vi "keyboardInput.vi"() -> ()   [LabVIEW 2023]
uses:
  <vilib>/regexp/Match Regular Expression.xnode
panel:
  out "Waveform Chart":dbl(graph)
  in  "MAIN STOP":bool
  out "data out 2":string
  out "code 2":i32
  in  "stop 4":bool
  out "Ostatnia 2":string
  out "PID":string
  in  "stop":bool
  in  "stop 3":bool
  out "code":i32
  out "Ostatnia":string
  out "data out":string
  in  "stop 2":bool
  out "ASCII Char 2":i16
  out "Character 2":string
  out "standard output 2":string
  out "standard output":string
  out "Character":string
  out "ASCII Char":i16
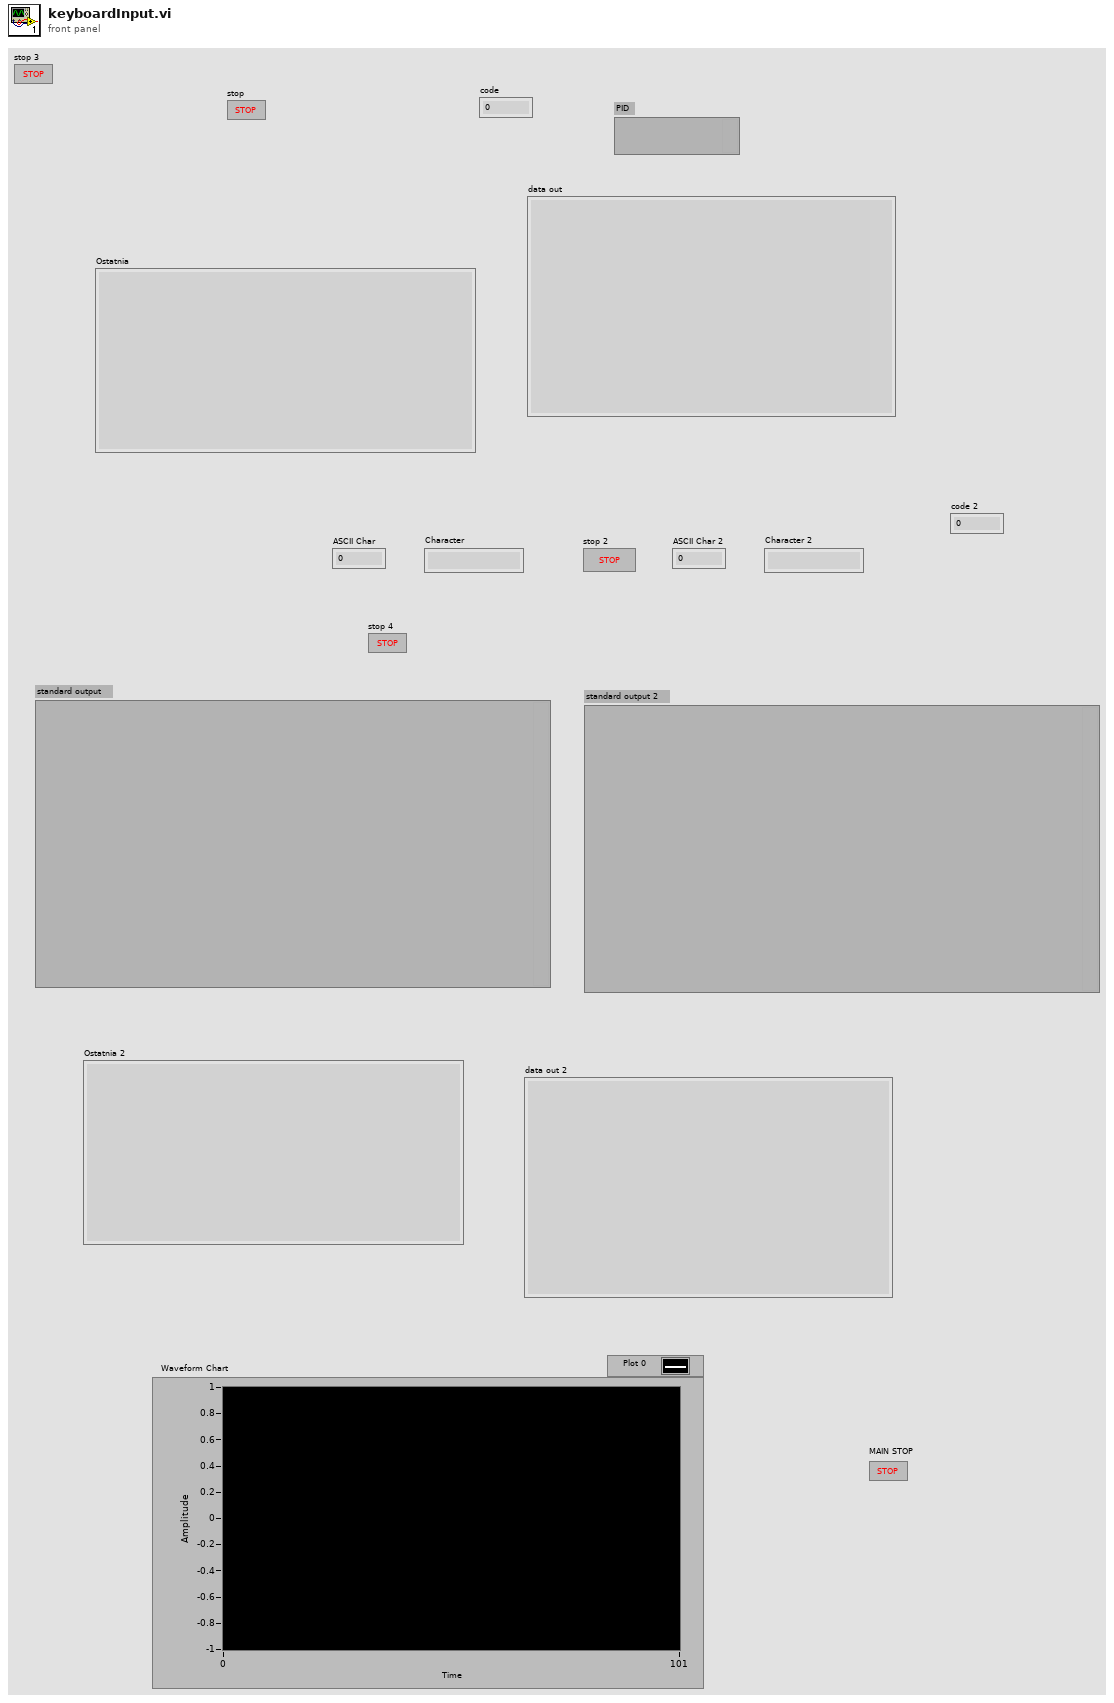
[diagram p1: front panel]
types:
  T1 = enum16{"Standard", "Buffered", "CRLF", "Immediate"}
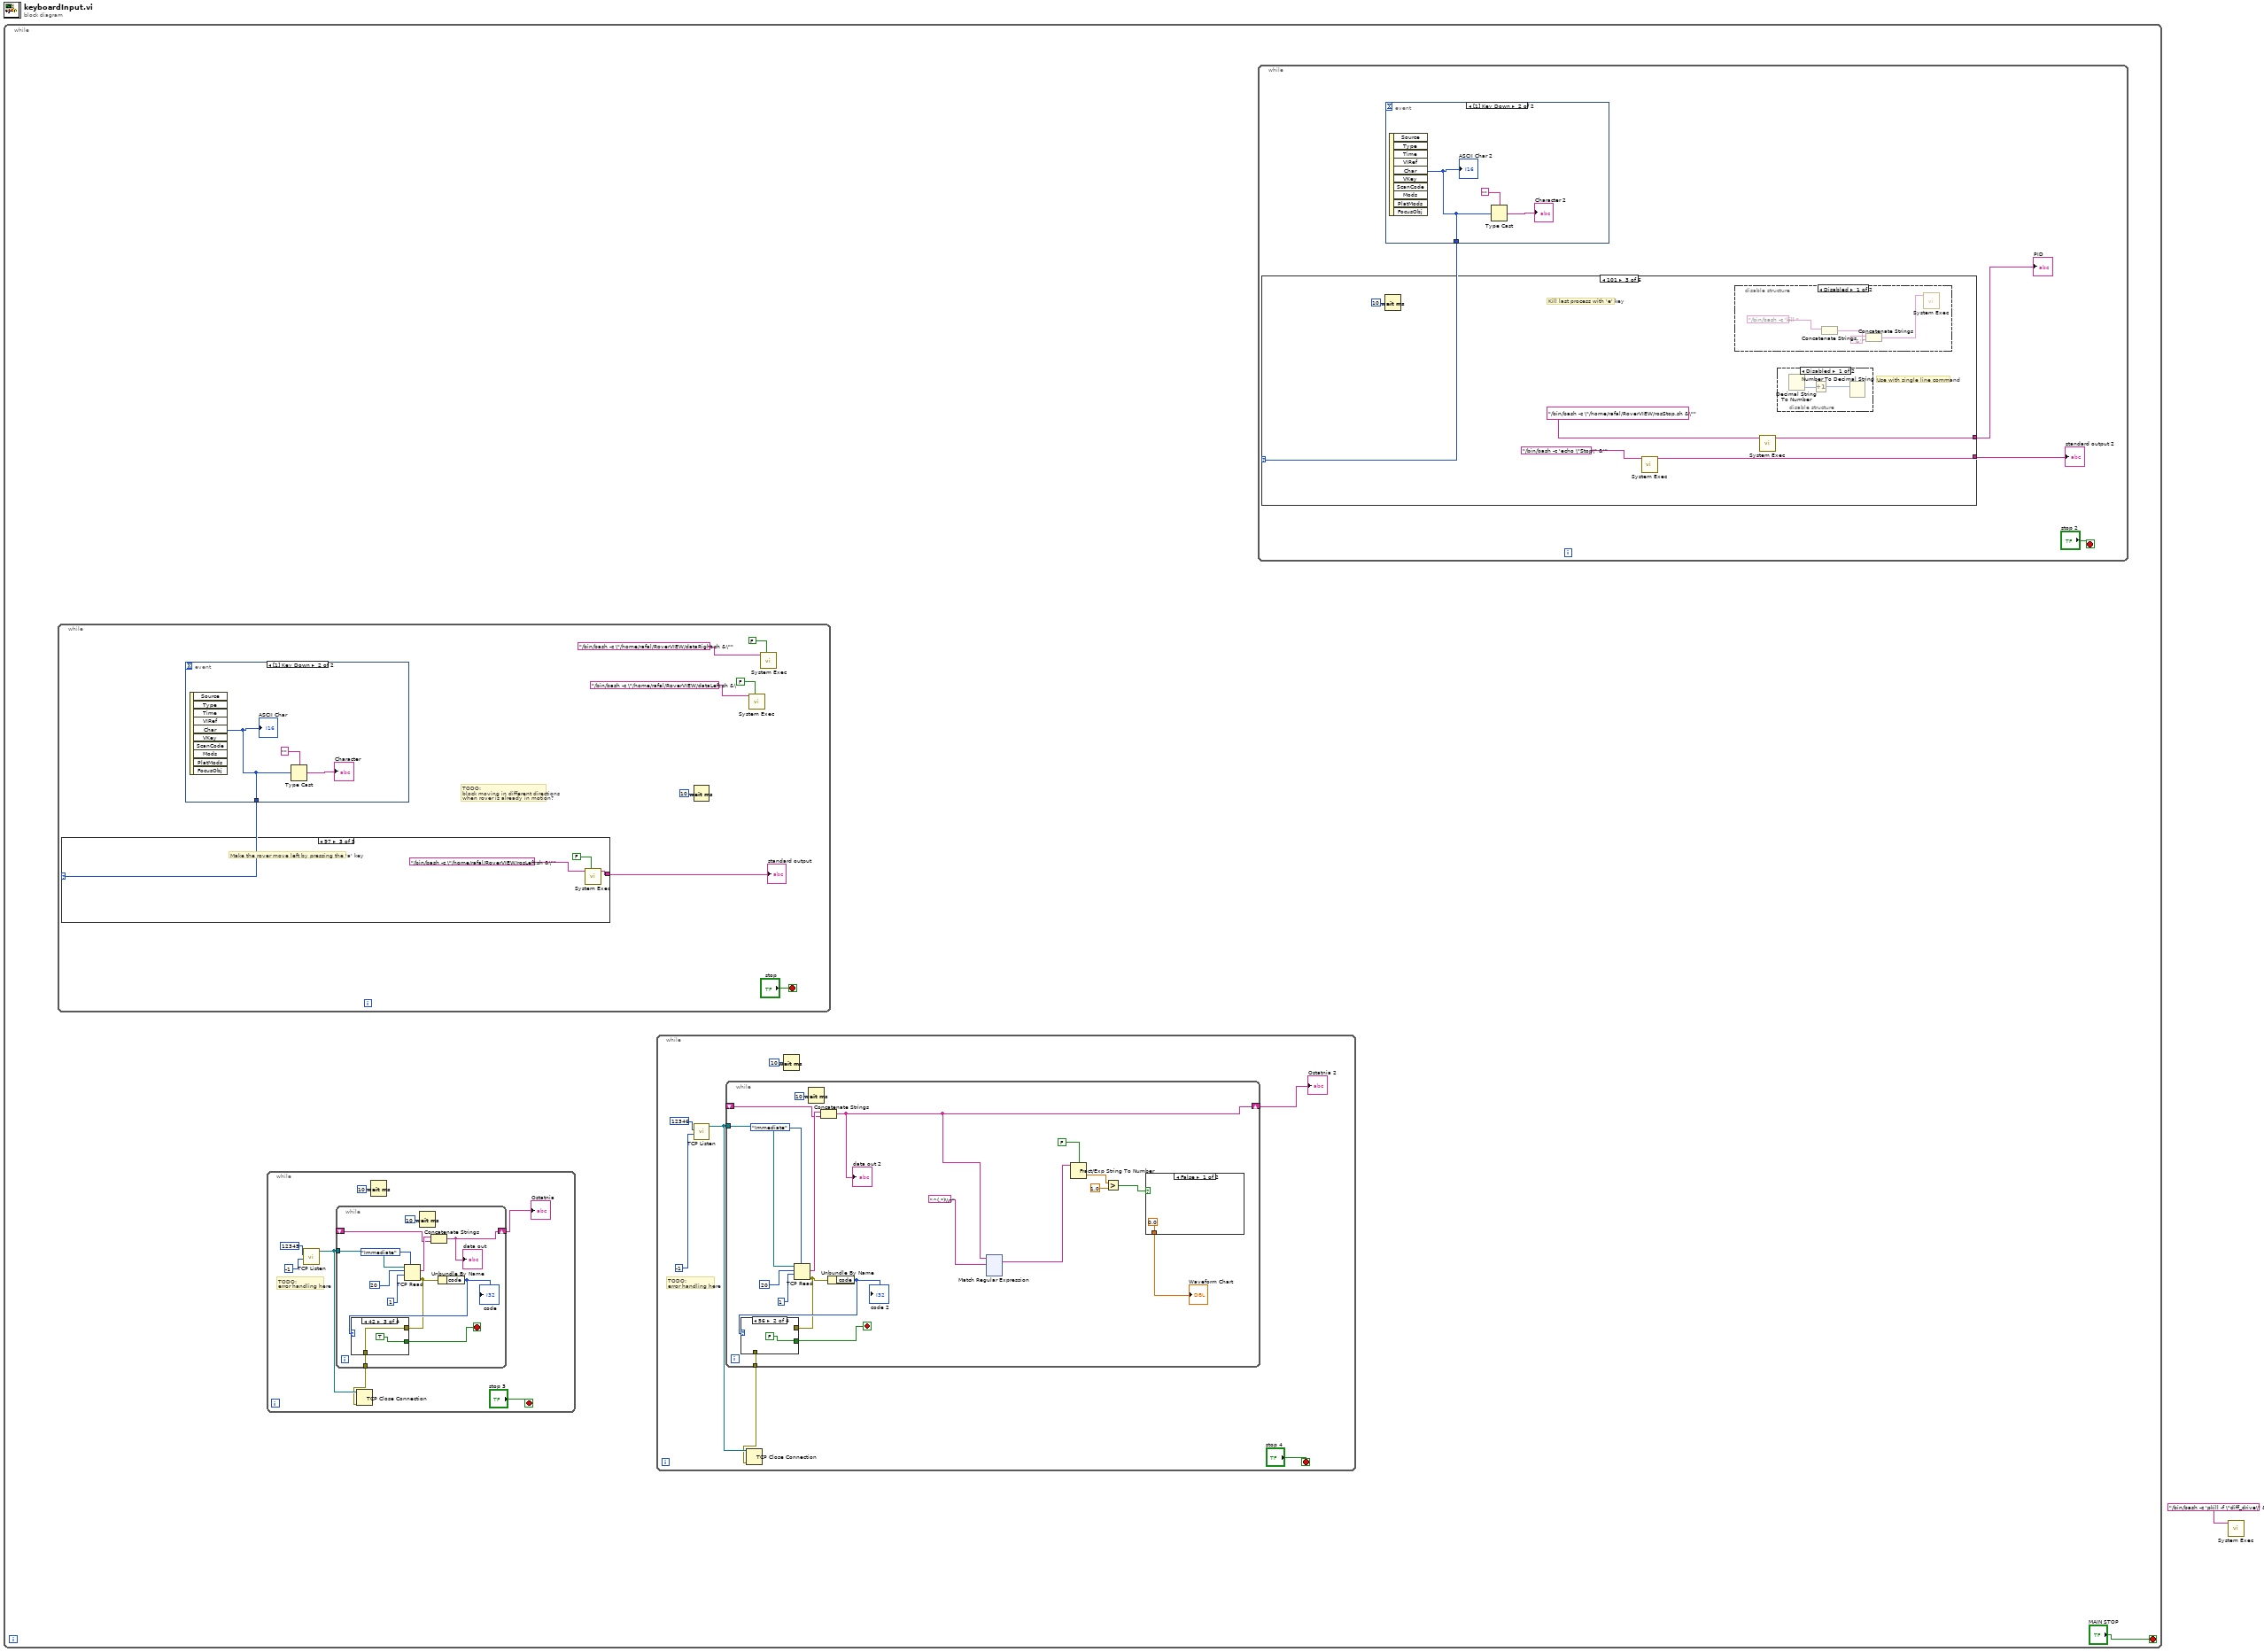
[diagram p0: block diagram]
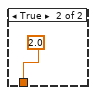
[diagram p2: hidden frame]
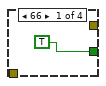
[diagram p3: hidden frame]
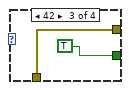
[diagram p4: hidden frame]
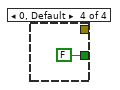
[diagram p5: hidden frame]
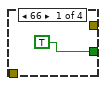
[diagram p6: hidden frame]
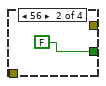
[diagram p7: hidden frame]
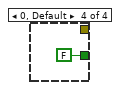
[diagram p8: hidden frame]
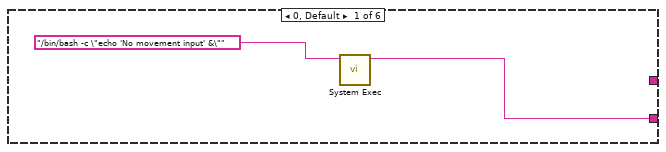
[diagram p9: hidden frame]
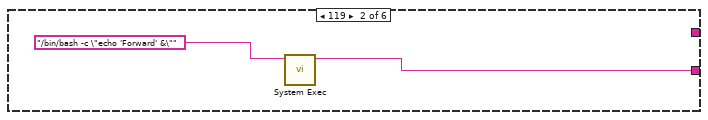
[diagram p10: hidden frame]
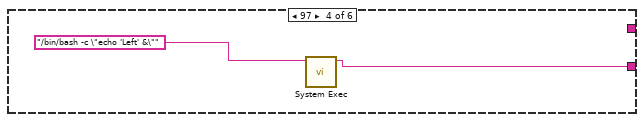
[diagram p13: hidden frame]
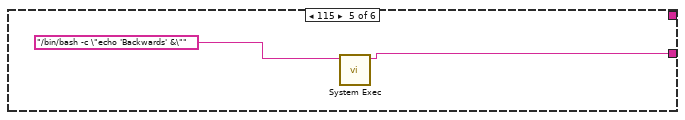
[diagram p14: hidden frame]
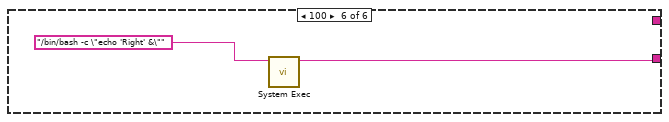
[diagram p15: hidden frame]
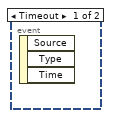
[diagram p16: hidden frame]
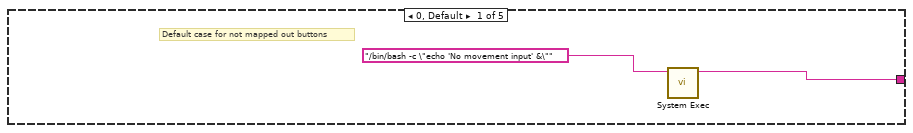
[diagram p17: hidden frame]
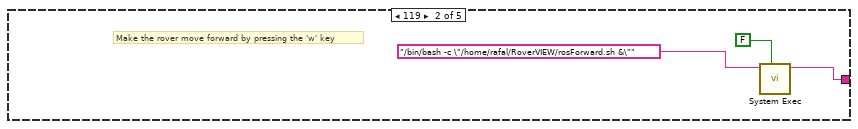
[diagram p18: hidden frame]
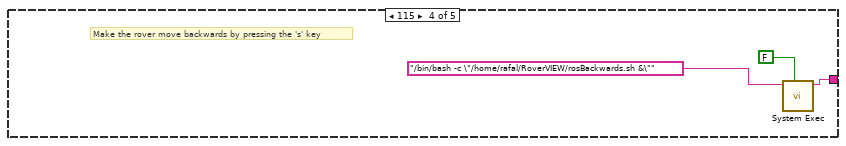
[diagram p19: hidden frame]
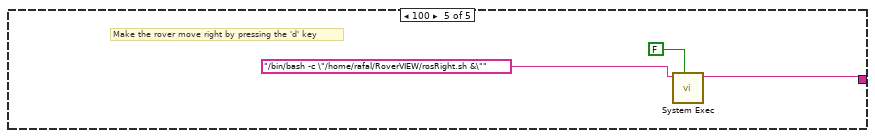
[diagram p20: hidden frame]
diagram:
  n1 = while {
    stop <- "MAIN STOP" stop-if-true
    n2 = while {
      stop <- "stop" stop-if-true
      # "TODO: \nblock moving in different directions\nwhen rover is already in motion?"
      n3 = event shown="[1] Key Down" {
        selector: _ -> [_ _]
        dyn-events: _ -> [_ _]
        timeout: _ -> [_ _]
        tunnel: [_ w227] -> w212
        event Timeout {
          n4 = event-data() -> ()  [unwired: 1 in, 3 out]
        }
        event Key Down {
          n5 = event-data() -> ("Char"=w227:i16)  [unwired: 1 in, 9 out]
          "ASCII Char" <- w227
          n6 = Type Cast(type="", x=w227) -> (*(type *) &x=→"Character":string)
        }
      }
      n7 = case shown="97" w212 {
        tunnel: [w213 w216 w219 w222 w225] -> w211
        frame 0, Default {
          # "Default case for not mapped out buttons"
          n8 = call <vilib>:"System Exec.vi"("command line"="/bin/bash -c \"echo 'No movement input' &\"") -> ("standard output"=w213:string)  [unwired: 7 in, 3 out]
        }
        frame 119 {
          # "Make the rover move forward by pressing the 'w' key"
          n9 = call <vilib>:"System Exec.vi"("wait until completion? (T)"=FALSE, "command line"="/bin/bash -c \"/home/rafal/RoverVIEW/rosForward.sh &\"") -> ("standard output"=w216:string)  [unwired: 6 in, 3 out]
        }
        frame 97 {
          # "Make the rover move left by pressing the 'a' key"
          n10 = call <vilib>:"System Exec.vi"("wait until completion? (T)"=FALSE, "command line"="/bin/bash -c \"/home/rafal/RoverVIEW/rosLeft.sh &\"") -> ("standard output"=w219:string)  [unwired: 6 in, 3 out]
        }
        frame 115 {
          # "Make the rover move backwards by pressing the 's' key"
          n11 = call <vilib>:"System Exec.vi"("wait until completion? (T)"=FALSE, "command line"="/bin/bash -c \"/home/rafal/RoverVIEW/rosBackwards.sh &\"") -> ("standard output"=w222:string)  [unwired: 6 in, 3 out]
        }
        frame 100 {
          # "Make the rover move right by pressing the 'd' key"
          n12 = call <vilib>:"System Exec.vi"("wait until completion? (T)"=FALSE, "command line"="/bin/bash -c \"/home/rafal/RoverVIEW/rosRight.sh &\"") -> ("standard output"=w225:string)  [unwired: 6 in, 3 out]
        }
      }
      "standard output" <- w211
      n13 = Wait (ms)(milliseconds to wait=u32 10) -> ()  [unwired: 1 out]
      n14 = call <vilib>:"System Exec.vi"("wait until completion? (T)"=FALSE, "command line"="/bin/bash -c \"/home/rafal/RoverVIEW/dataLeft.sh &\"") -> ()  [unwired: 6 in, 4 out]
      n15 = call <vilib>:"System Exec.vi"("wait until completion? (T)"=FALSE, "command line"="/bin/bash -c \"/home/rafal/RoverVIEW/dataRight.sh &\"") -> ()  [unwired: 6 in, 4 out]
    }
    n16 = while {
      stop <- "stop 3" stop-if-true
      # "TODO:\nerror handling here"
      n17 = call <vilib>:"TCP Listen.vi"("timeout ms (wait forever: -1)"=-1, "port"=u16 12345) -> ("connection ID"=w159:refnum<k5>)  [unwired: 5 in, 4 out]
      n18 = while {
        tunnel: w159 -> [w169]
        shift-right: [w166] -> w154
        shift-left: _ -> [w167]
        tunnel: [w162] -> w156
        stop <- w164 stop-if-true
        n19 = TCP Read(connection ID=w169, bytes to read=20, 7:T1."Immediate" ("mode (standard)"), 9:1 ("timeout ms (25000)")) -> (data out=w168:string, error out=w163:errorcluster)  [unwired: 1 in, 1 out]
        n20 = Wait (ms)(milliseconds to wait=u32 10) -> ()  [unwired: 1 out]
        n21 = Concatenate Strings(w168, w167) -> (w166:string)
        "data out" <- w166
        n22 = Unbundle By Name(w163) -> ("code"=w165:i32)
        "code" <- w165
        n23 = case shown="42" w165 {
          tunnel: [TRUE FALSE TRUE FALSE] -> w164
          tunnel: w163 -> [_ _ w174 _]
          tunnel: [_ _ w174 _] -> w162
          frame 66 {
          }
          frame 56 {
          }
          frame 42 {
          }
          frame 0, Default {
          }
        }
      }
      "Ostatnia" <- w154
      n24 = TCP Close Connection(connection ID=w159, error in (no error)=w156) -> ()  [unwired: 1 in, 2 out]
      n25 = Wait (ms)(milliseconds to wait=u32 10) -> ()  [unwired: 1 out]
    }
    n26 = while {
      stop <- "stop 4" stop-if-true
      # "TODO:\nerror handling here"
      n27 = call <vilib>:"TCP Listen.vi"("timeout ms (wait forever: -1)"=-1, "port"=u16 12346) -> ("connection ID"=w9:refnum<k5>)  [unwired: 5 in, 4 out]
      n28 = while {
        tunnel: w9 -> [w26]
        shift-right: [w14] -> w3
        shift-left: _ -> [w24]
        tunnel: [w20] -> w6
        stop <- w22 stop-if-true
        n29 = TCP Read(connection ID=w26, bytes to read=20, 7:T1."Immediate" ("mode (standard)"), 9:1 ("timeout ms (25000)")) -> (data out=w25:string, error out=w21:errorcluster)  [unwired: 1 in, 1 out]
        n30 = Wait (ms)(milliseconds to wait=u32 10) -> ()  [unwired: 1 out]
        n31 = Concatenate Strings(w25, w24) -> (w14:string)
        "data out 2" <- w14
        n32 = Unbundle By Name(w21) -> ("code"=w23:i32)
        "code 2" <- w23
        n33 = case shown="56" w23 {
          tunnel: [TRUE FALSE TRUE FALSE] -> w22
          tunnel: w21 -> [_ _ w150 _]
          tunnel: [_ _ w150 _] -> w20
          frame 66 {
          }
          frame 56 {
          }
          frame 42 {
          }
          frame 0, Default {
          }
        }
        n34 = xnode "Match Regular Expression"("input string"=w14, "regular expression"="^(.*)\\n") -> ("whole match"=w17:string)  [unwired: 4 in, 4 out]
        n35 = Fract/Exp String To Number(use system decimal point (T)=FALSE, string=w17) -> (number=w11:dbl)  [unwired: 2 in, 1 out]
        n36 = Greater?(x=w11, y=1.0) -> (0:w13:bool)
        n37 = case shown="False" w13 {
          tunnel: [0.0 2.0] -> w10
          frame False {
          }
          frame True {
          }
        }
        "Waveform Chart" <- w10
      }
      "Ostatnia 2" <- w3
      n38 = TCP Close Connection(connection ID=w9, error in (no error)=w6) -> ()  [unwired: 1 in, 2 out]
      n39 = Wait (ms)(milliseconds to wait=u32 10) -> ()  [unwired: 1 out]
    }
    n40 = while {
      stop <- "stop 2" stop-if-true
      n41 = event shown="[1] Key Down" {
        selector: _ -> [_ _]
        dyn-events: _ -> [_ _]
        timeout: _ -> [_ _]
        tunnel: [_ w202] -> w179
        event Timeout {
          n42 = event-data() -> ()  [unwired: 1 in, 3 out]
        }
        event Key Down {
          n43 = event-data() -> ("Char"=w202:i16)  [unwired: 1 in, 9 out]
          "ASCII Char 2" <- w202
          n44 = Type Cast(type="", x=w202) -> (*(type *) &x=→"Character 2":string)
        }
      }
      n45 = case shown="101" w179 {
        tunnel: [w181 w183 w188 w196 w198 w200] -> w178
        tunnel: [_ _ w187 _ _ _] -> w177
        frame 0, Default {
          n46 = call <vilib>:"System Exec.vi"("command line"="/bin/bash -c \"echo 'No movement input' &\"") -> ("standard output"=w181:string)  [unwired: 7 in, 3 out]
        }
        frame 119 {
          n47 = call <vilib>:"System Exec.vi"("command line"="/bin/bash -c \"echo 'Forward' &\"") -> ("standard output"=w183:string)  [unwired: 7 in, 3 out]
        }
        frame 101 {
          # "Use with single line command"
          # "Kill last process with 'e' key"
          n48 = Wait (ms)(milliseconds to wait=u32 10) -> ()  [unwired: 1 out]
          n49 = call <vilib>:"System Exec.vi"("command line"="/bin/bash -c 'echo \"Stop\" &'") -> ("standard output"=w188:string)  [unwired: 7 in, 3 out]
          n50 = disable-structure shown="Disabled" {
            frame Disabled {
              n51 = Concatenate Strings("/bin/bash -c 'kill " ("string")) -> (w192:string)  [unwired: 1 in]
              n52 = Concatenate Strings(w192, " &'" ("string")) -> (w190:string)
              n53 = call <vilib>:"System Exec.vi"("command line"=w190) -> ()  [unwired: 7 in, 4 out]
            }
            frame Enabled {
            }
          }
          n54 = call <vilib>:"System Exec.vi"("command line"="/bin/bash -c \"/home/rafal/RoverVIEW/rosStop.sh &\"") -> ("standard output"=w187:string)  [unwired: 7 in, 3 out]
          n55 = disable-structure shown="Disabled" {
            frame Disabled {
              n56 = Decimal String To Number() -> (number=w194:i32)  [unwired: 3 in, 1 out]
              n57 = Increment(x=w194) -> (x+1=w195:i32)
              n58 = Number To Decimal String(number=w195) -> ()  [unwired: 1 in, 1 out]
            }
            frame Enabled {
            }
          }
        }
        frame 97 {
          n59 = call <vilib>:"System Exec.vi"("command line"="/bin/bash -c \"echo 'Left' &\"") -> ("standard output"=w196:string)  [unwired: 7 in, 3 out]
        }
        frame 115 {
          n60 = call <vilib>:"System Exec.vi"("command line"="/bin/bash -c \"echo 'Backwards' &\"") -> ("standard output"=w198:string)  [unwired: 7 in, 3 out]
        }
        frame 100 {
          n61 = call <vilib>:"System Exec.vi"("command line"="/bin/bash -c \"echo 'Right' &\"") -> ("standard output"=w200:string)  [unwired: 7 in, 3 out]
        }
      }
      "standard output 2" <- w178
      "PID" <- w177
    }
  }
  n62 = call <vilib>:"System Exec.vi"("command line"="/bin/bash -c 'pkill -f \"diff_drive\" &'") -> ()  [unwired: 7 in, 4 out]
